vi "ChannelDecode.vi"(8 "error in (no error)":errorcluster, 10 "Code Cluster":T1={"Code type"=enum."No code", "Encode factor"=2, "Constraint length(For convolution code)"=3}, 11 "Received bits":i8[](array[numeric])) -> (0 "error out":errorcluster, 3 "Decoded bits":i8[](array[numeric]))   [LabVIEW 2014]
panel:
  out "size(s) 2":i32
  out "size(s)":i32
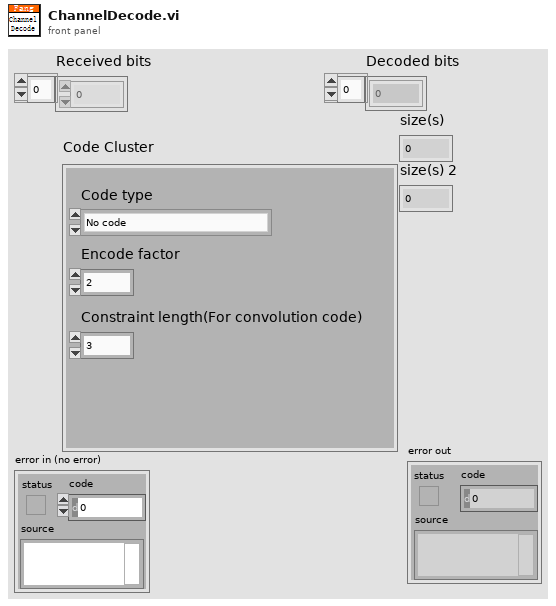
[diagram p1: front panel]
types:
  T1 = cluster{"Code type":enum16{"No code", "Convolution code", "Repetition code", "TD-Repetition code"}, "Encode factor":i32, "Constraint length(For convolution code)":i32}
  T2 = enum16{"No code", "Convolution code", "Repetition code", "TD-Repetition code"}
  T3 = cluster{"constraint length (K)":i32, "initial state":u32, "Encode factor":i32}
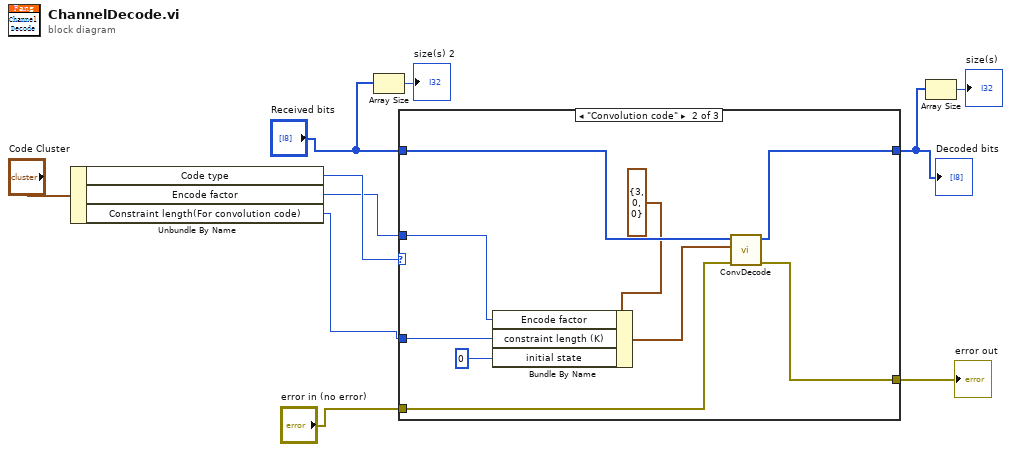
[diagram p0: block diagram]
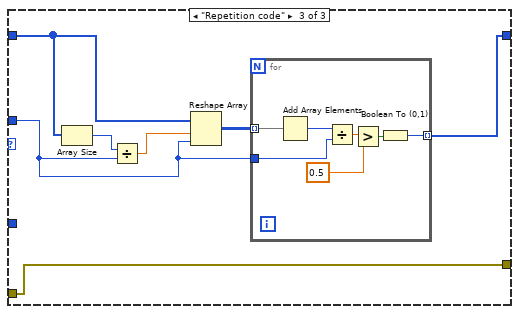
[diagram p3: hidden frame]
diagram:
  n1 = Unbundle By Name("Code Cluster") -> ("Code type"=w9:T2, "Encode factor"=w7:i32, "Constraint length(For convolution code)"=w8:i32)
  n2 = Array Size(array="Received bits") -> (size(s)=→"size(s) 2":i32)
  n3 = case shown="\"Convolution code\"" w9 {
    tunnel: "Received bits" -> [w12 w21 w28]
    tunnel: [w12 w13 w23] -> w4
    tunnel: w8 -> [_ w19 _]
    tunnel: w7 -> [_ w17 w24]
    tunnel: "error in (no error)" -> [w11 w15 w22]
    tunnel: [w11 w14 w22] -> w5
    frame "No code", Default {
    }
    frame "Convolution code" {
      n4 = Bundle By Name(cluster=T3 {"constraint length (K)"=3, "initial state"=0, "Encode factor"=0} ("Decode Parameter"), "Encode factor"=w17, "constraint length (K)"=w19, "initial state"=u32 0) -> (w16:T3)
      n5 = call "ConvDecode.vi"("error in (no error)"=w15, "Encode Parameter"=w16, "Input Bits"=w21) -> ("error out"=w14:errorcluster, "output bit stream"=w13:i8[])  [unwired: 7 in]
    }
    frame "Repetition code" {
      n6 = Array Size(array=w28) -> (size(s)=w27:i32)
      n7 = Divide(x=w27, y=w24) -> (x/y=w26:dbl)
      n8 = Reshape Array(w28, w26, w24) -> (w25:i8[][])
      n9 = for {
        tunnel: w25 -> [w35] mode=indexing
        tunnel: w24 -> [w33]
        tunnel: [w29] -> w23 mode=indexing
        n10 = Add Array Elements(numeric array=w35) -> (sum=w34:i8)
        n11 = Divide(x=w34, y=w33) -> (x/y=w32:dbl)
        n12 = Greater?(x=w32, y=0.5) -> (0:w30:bool)
        n13 = Boolean To (0,1)(Boolean=w30) -> (0, 1=w29:i16)
      }
    }
  }
  "Decoded bits" <- w4
  "error out" <- w5
  n14 = Array Size(array=w4) -> (size(s)=→"size(s)":i32)
